vi "ief_get_state.vi"(0 "Tagprefix in":refnum<k21>, 1 "error in (no error)":errorcluster) -> (2 "Tagprefix out":refnum<k21>, 3 "PA State":u8, 4 "error out (no error)":errorcluster)   [LabVIEW 2015, in "IEF Werner.lvlib"]
doc: "The VI returns the present PA control state.\n\nPA Control State Range:\n01, hex - basic mode\n02, hex - manual mode\n10, hex - automatik mode started\n11, hex - automatic mode\n12, hex - automatic mode, stop recognized \n13, hex - automatic mode, stop program in progress\n15, hex - automatic mode, stopped\n16, hex - automatic mode, program start to stop running\n17, hex - automatic mode, error recognized\n18, hex - automatic mode, error program in progress\n19, hex - automatic mode, error and stopped\n20, hex - manual mode, serial\n30, hex - online mode, started\n31, hex - online mode\n32, hex - online mode, stop recognized\n35, hex - online mode, stopped\n37, hex - online mode, error recognized\n39, hex - online mode, error recognized and stopped"
uses:
  IEF Werner.lvlib
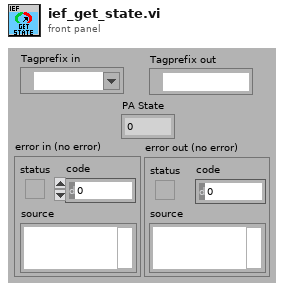
[diagram p1: front panel]
types:
  T1 = typedef "Semaphore RefNum" = refnum<k1>
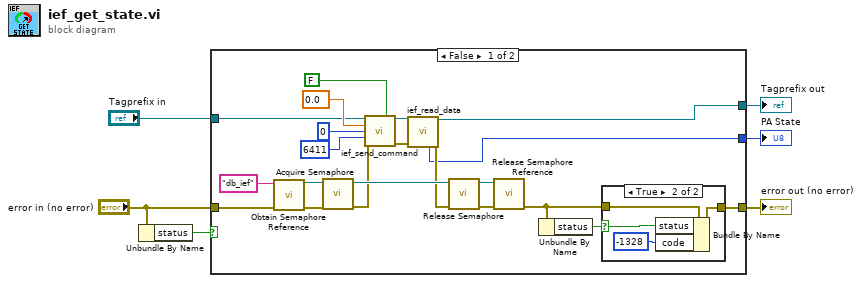
[diagram p0: block diagram]
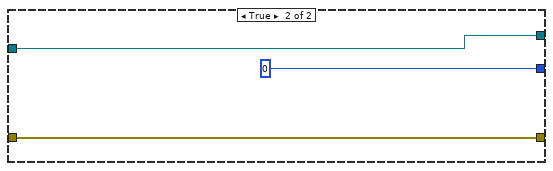
[diagram p3: hidden frame]
diagram:
  n1 = Unbundle By Name("error in (no error)") -> ("status"=w4:bool)
  n2 = case shown="False" w4 {
    tunnel: "error in (no error)" -> [w17 w35]
    tunnel: [w24 w35] -> w6
    tunnel: [w7 u16 0 ("value uint 16")] -> w3
    tunnel: "Tagprefix in" -> [w10 w34]
    tunnel: [w8 w34] -> w1
    frame False {
      n3 = call <vilib>:"Obtain Semaphore Reference.vi"("error in (no error)"=w17, "name (unnamed)"="db_ief") -> ("error out"=w21:errorcluster, "semaphore"=w22:T1)  [unwired: 3 in, 1 out]
      n4 = call <vilib>:"Acquire Semaphore.vi"("error in (no error)"=w21, "semaphore"=w22) -> ("error out"=w16:errorcluster, "semaphore out"=w20:T1)  [unwired: 3 in, 1 out]
      n5 = call "ief_send_command.vi"("Tagprefix in"=w10, "Command datum of type real"=FALSE, "Command datum"=sgl 0.0, "Command parameter"=u16 0, "Command code"=u16 6411, "error in (no error)"=w16) -> ("Tagprefix out"=w9:refnum<k21>, "error out (no error)"=w25:errorcluster)  [unwired: 4 in, 4 out]
      n6 = call "ief_read_data.vi"("Tagprefix in"=w9, "error in (no error)"=w25) -> ("Tagprefix out"=w8:refnum<k21>, "PA Control state"=w7:u8, "error out (no error)"=w15:errorcluster)  [unwired: 7 in, 4 out]
      n7 = call <vilib>:"Release Semaphore.vi"("error in (no error)"=w15, "semaphore"=w20) -> ("error out"=w19:errorcluster, "semaphore out"=w18:T1)  [unwired: 4 in]
      n8 = call <vilib>:"Release Semaphore Reference.vi"("error in (no error)"=w19, "semaphore"=w18) -> ("error out"=w14:errorcluster)  [unwired: 8 in, 1 out]
      n9 = Unbundle By Name(w14) -> ("status"=w11:bool)
      n10 = case shown="True" w11 {
        selector: w11 -> [_ w29]
        tunnel: [w28 w31] -> w24
        tunnel: w14 -> [w28 w32]
        frame False {
        }
        frame True {
          n11 = Bundle By Name(cluster=w32, "status"=w29, "code"=-1328) -> (w31:errorcluster)
        }
      }
    }
    frame True {
    }
  }
  "error out (no error)" <- w6
  "PA State" <- w3
  "Tagprefix out" <- w1
